vi "COMI US Retrv One.vi"(9 "scanCount":u32, 10 "chOrder":i32, 11 "hDevice":u32) -> (2 "function return":i16, 3 "hDevice out":u32)   [LabVIEW 2017, in "Comidll.lvlib"]
doc: "short (COMI_US_RetrvOne) (HANDLE hDevice, int chOrder, unsigned long scanCount);"
uses:
  <userlib>/Comidll/Comidll.lvlib
  <userlib>/Comidll/Comidll.dll
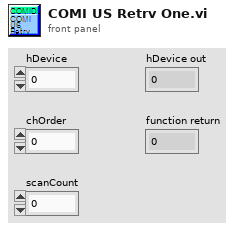
[diagram p1: front panel]
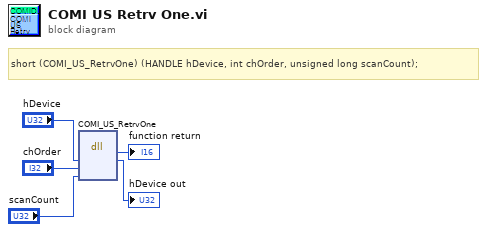
[diagram p0: block diagram]
diagram:
  # "short\t(COMI_US_RetrvOne) (HANDLE hDevice, int chOrder, unsigned long scanCount);"
  n1 = dll-call lib="C:/Program Files/National Instruments/LabVIEW 2017/user.lib/Comidll/Comidll.*" fn="COMI_US_RetrvOne"("hDevice"="hDevice", "chOrder"="chOrder", "scanCount"="scanCount") -> (→"function return":i16, "hDevice"=→"hDevice out":u32)  [unwired: 5 in, 2 out]
